vi "execution class name.vi"(8 "error in":errorcluster, 11 "configuration in":refnum<class "base TBM sequencer configuration.lvclass">) -> (0 "error out":errorcluster, 2 "execution class":string, 3 "configuration out":refnum<class "base TBM sequencer configuration.lvclass">)   [LabVIEW 2015, in "base TBM sequencer configuration.lvclass"]
uses:
  base TBM sequencer configuration.lvclass
  <vilib>/NI/Tag Bus Module Framework/module configuration/TBM module configuration.lvclass
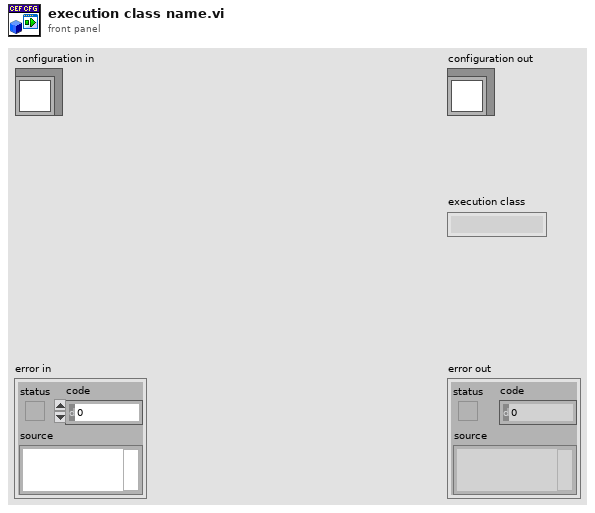
[diagram p1: front panel]
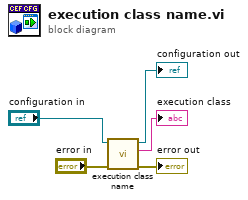
[diagram p0: block diagram]
diagram:
  n1 = call-parent "execution class name.vi"("error in"="error in", "configuration in"="configuration in") -> ("error out"=→"error out":errorcluster, "execution class"=→"execution class":string, "configuration out"=→"configuration out":refnum<class "base TBM sequencer configuration.lvclass">)  [unwired: 7 in]
